vi "FTW-Logger-Launch.vi"(5 "FTW Logger Configuration":string="{\n  \"Identity\": \"EventLog\",\n  \"InboxAddress\": \"lvq://*\",\n  \"PublisherAddress\": \"\",\n  \"LoggerAddress\": \"\",\n  \"DebugEnableInboxLogging\": false,\n  \"DebugEnableJobLogging\": false,\n  \"DebugShowPanel\": false,\n  \"ApplicationName\": \"Featherweight Application\",\n  \"LoggerName\": \"Log\",\n  \"LoggerDirectory\": \"[UserAppDir]\\\\Featherweight\\\\Logs\",\n  \"LoggerDiskThrashDelay\": 200\n}", 11 "error in":errorcluster) -> (4 "FTW Logger Connector":refnum<class "FTW-Logger.lvclass">, 6 "Logger Address":string, 15 "error out":errorcluster)   [LabVIEW 2013, in "FTW-Actor.lvlib" / "FTW-Logger.lvclass"]
doc: "This method launches a Logger Process which is then referred to based on its LoggerID. Normally in a LabVIEW application, an object's methods would adhere to dataflow with the object wired to the method; however, the Logger Process object likely needs to be accessed by many different portions of your application, and for this reason, it is called by reference, where the LoggerID string refers to the logger.\n\nThis method should be called as one of the very first actions in your application to reasonably ensure the buffer of logged events does not overflow. Events that are logged prior to launching the Logger Process with this method are queued, and will be logged once this process begins."
uses:
  FTW-Logger.lvclass
  Core/FTW-Logger-Process.vi
  Connector/FTW-ActorConnector.lvclass
  Core/FTW-Logger-Core.lvclass
panel:
  # "Inputs"
  # "Outputs"
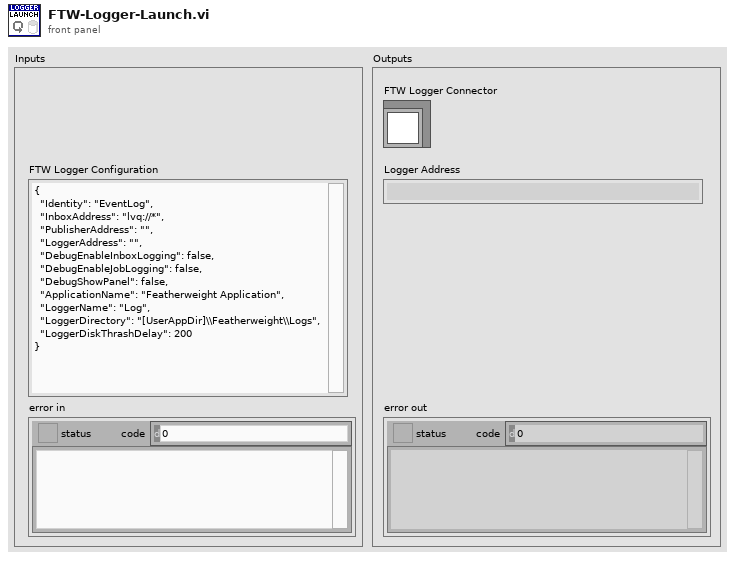
[diagram p1: front panel]
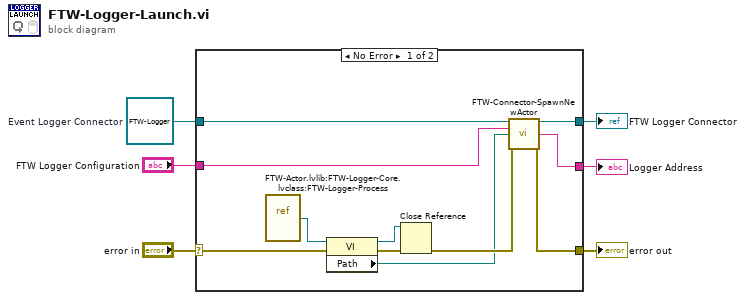
[diagram p0: block diagram]
diagram:
  w3 = refnum<class "FTW-Logger.lvclass"> refnum  # Event Logger Connector
  n1 = case shown="No Error" "error in" {
    selector: "error in" -> [w9 w19]
    tunnel: [w14 w19] -> w6
    tunnel: [w15 w18] -> w4
    tunnel: w3 -> [w17 w18]
    tunnel: "FTW Logger Configuration" -> [w16 _]
    tunnel: [w13 _] -> w1
    frame No Error {
      n2 = vi-ref "FTW-Actor.lvlib:FTW-Logger-Core.lvclass:FTW-Logger-Process.vi"() -> (w12:refnum<vi>)
      n3 = property class="VI"(reference=w12, error in=w9) -> (reference out=w11:refnum<vi>, error out=w10:errorcluster, "Path"=w7:path)
      n4 = Close Reference(reference=w11, error in (no error)=w10) -> (error out=w8:errorcluster)
      n5 = call "FTW-Connector-SpawnNewActor.vi"("FTW Actor Connector Type"=w17, "Configuration"=w16, "Actor VI Filepath"=w7, "error in"=w8) -> ("FTW Actor Connector"=w15:refnum<class "FTW-Logger.lvclass">, "Instance Inbox Address"=w13:string, "error out"=w14:errorcluster)  [unwired: 7 in, 2 out]
    }
    frame Error {
    }
  }
  "error out" <- w6
  "FTW Logger Connector" <- w4
  "Logger Address" <- w1
